vi "Find Resource by Type (I32).vi"(10 "Resource Type":u32, 11 "Resources":T2) -> (1 "Index":i32, 2 "Found?":bool, 3 "Resource":T1)   [LabVIEW 2019]
uses:
  <resource>/dialog/QuickDrop/plugins/PaneRelief/Low-Level VI Manipulation/Resource Array.ctl
  <resource>/dialog/QuickDrop/plugins/PaneRelief/Low-Level VI Manipulation/Resource.ctl
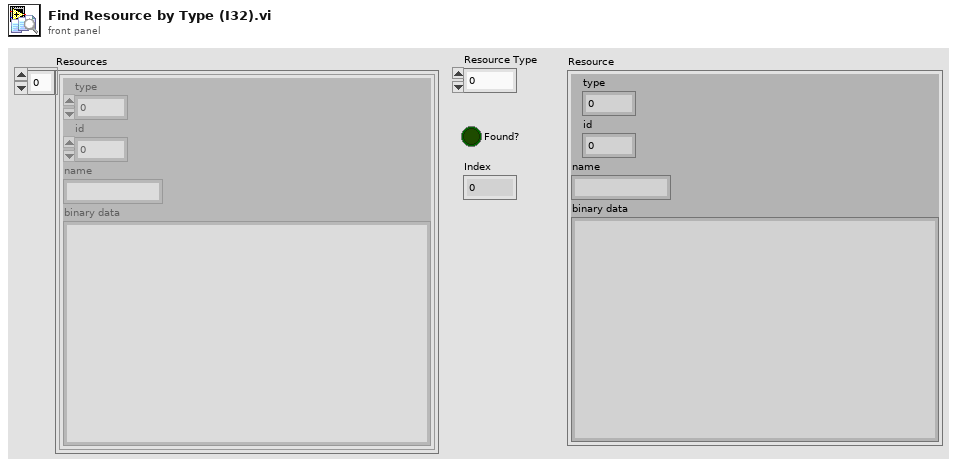
[diagram p1: front panel]
types:
  T1 = typedef "Resource.ctl" = cluster{"type":u32, "id":i32, "name":string, "binary data":string}
  T2 = typedef "Resource Array.ctl" = T1[]
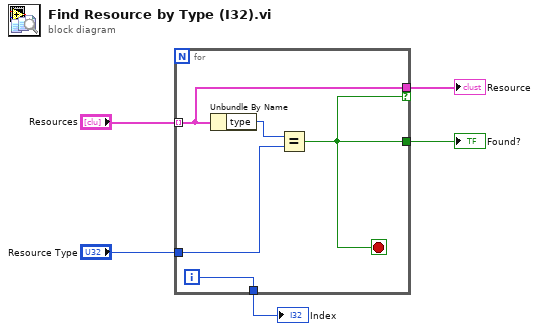
[diagram p0: block diagram]
diagram:
  n1 = for {
    tunnel: "Resources" -> [w8] mode=indexing
    tunnel: "Resource Type" -> [w9]
    tunnel: [w7] -> w3
    tunnel: [w8] -> w2 if=w7
    tunnel: [w6] -> w1
    i -> [w6]
    stop <- w7 stop-if-true
    n2 = Unbundle By Name(w8) -> ("type"=w10:u32)
    n3 = Equal?(x=w10, y=w9) -> (x = y?=w7:bool)
  }
  "Resource" <- w2
  "Found?" <- w3
  "Index" <- w1
